vi "Counter_down.vi"(9 "load":bool, 10 "enable":bool=TRUE, 11 "limit":u16) -> (2 "count = 0?":bool, 3 "count":u16)   [LabVIEW 2017]
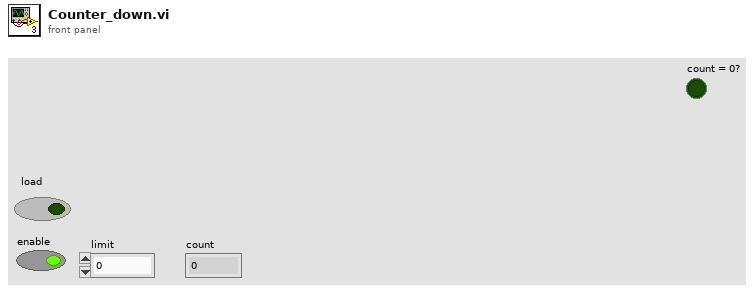
[diagram p1: front panel]
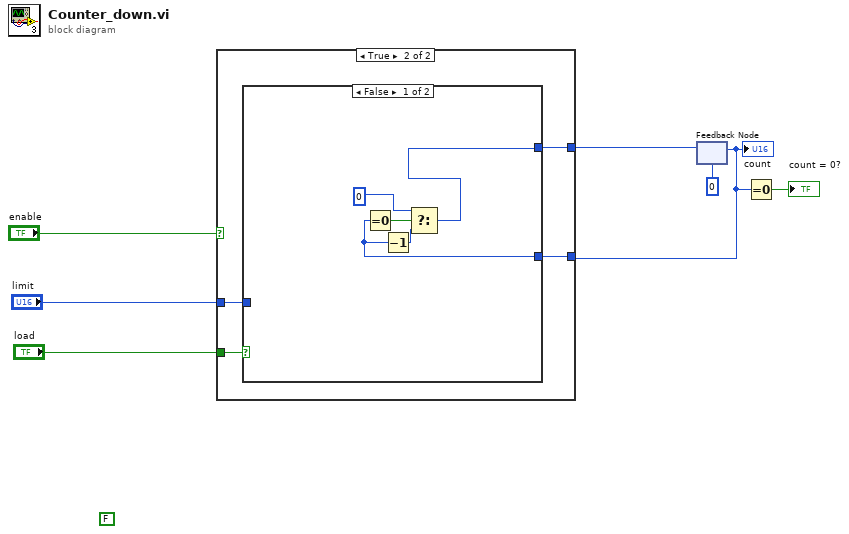
[diagram p0: block diagram]
diagram:
  (unwired) FALSE ("t")
  n1 = feedback #1(u16 0) -> (w2:u16)
  "count" <- w2
  n2 = case shown="True" "enable" {
    tunnel: "limit" -> [_ w12]
    tunnel: [w8 w11] -> w5
    tunnel: w2 -> [w8 w9]
    tunnel: "load" -> [_ w10]
    frame False {
    }
    frame True {
      n3 = case shown="False" w10 {
        tunnel: w12 -> [_ w18]
        tunnel: [w15 w18] -> w11
        tunnel: w9 -> [w13 _]
        frame False {
          n4 = Equal To 0?(x=w13) -> (x = 0?=w14:bool)
          n5 = Decrement(x=w13) -> (x-1=w16:u16)
          n6 = Select(t=u16 0, s=w14, f=w16) -> (s? t:f=w15:u16)
        }
        frame True {
        }
      }
    }
  }
  n7 = feedback-in #1(w5) -> ()
  n8 = Equal To 0?(x=w2) -> (x = 0?=→"count = 0?":bool)
